vi "deinitialize.vi"(0 "HGF_ThreadPool in":refnum<class "HGF_ThreadPool.lvclass">, 5 "error in (no error)":errorcluster) -> (19 "error out":errorcluster)   [LabVIEW 2014, in "HGF_BaseClasses.lvlib" / "HGF_ThreadPool.lvclass"]
doc: "This is a dynamic dispatch VI. It can be overwritten by childclasses to release allocated recources."
uses:
  HGF_ThreadPool.lvclass
  HGF_Base/HGF_Base.lvclass
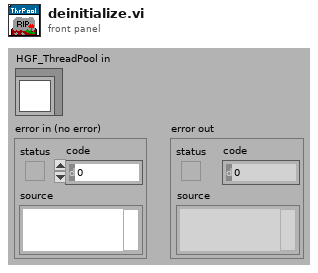
[diagram p1: front panel]
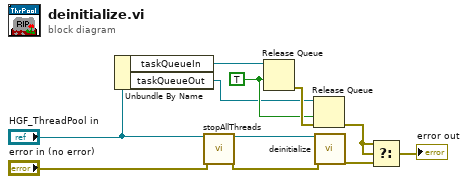
[diagram p0: block diagram]
diagram:
  w9 = TRUE ("force destroy? (F)")
  n1 = Unbundle By Name("HGF_ThreadPool in") -> ("taskQueueIn"=w11:refnum<queue>, "taskQueueOut"=w8:refnum<queue>)
  n2 = call "stopAllThreads.vi"("HGF_ThreadPool"="HGF_ThreadPool in", "error in (no error)"="error in (no error)") -> ("dup HGF_ThreadPool"=w2:refnum<class "HGF_ThreadPool.lvclass">, "error out"=w1:errorcluster)  [unwired: 16 out]
  n3 = Release Queue(queue=w11, force destroy? (F)=w9) -> (error out=w10:errorcluster)  [unwired: 1 in, 2 out]
  n4 = Release Queue(queue=w8, force destroy? (F)=w9, error in (no error)=w10) -> (error out=w7:errorcluster)  [unwired: 2 out]
  n5 = call-parent "deinitialize.vi"("HGF_Factory"=w2, "error in (no error)"=w1) -> ("error out"=w6:errorcluster)  [unwired: 17 out]
  n6 = Select(t=w7, s=w7, f=w6) -> (s? t:f=→"error out":errorcluster)
